vi "AO_equations_to_waveform.vi"(5 "variable/parameter names":string[](array[string]), 7 "minimum/current values":dbl[](array[numeric]), 8 "error in (no error)":errorcluster, 9 "Samples per second":dbl, 10 "Total AO Time":string, 11 "Analog Output Equations for each Channel":string[](array[string])) -> (0 "error out":errorcluster, 2 "Total # Samples":i32, 3 "Waveform Graph":waveform(dbl)[](graph))   [LabVIEW 2013]
uses:
  <vilib>/gmath/NI_Gmath.lvlib
  <vilib>/measure/NI_MAPro.lvlib
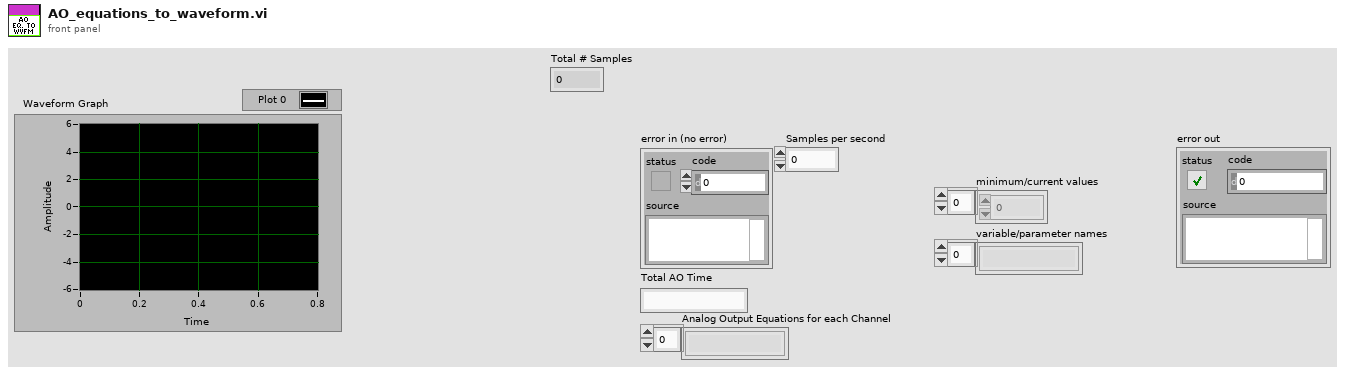
[diagram p1: front panel]
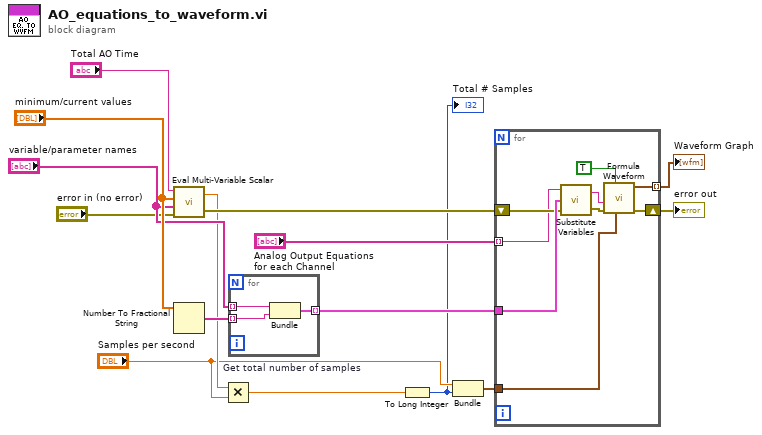
[diagram p0: block diagram]
diagram:
  n1 = call <vilib>:"Eval Multi-Variable Scalar.vi"("error in (no error)"="error in (no error)", "Variables"="variable/parameter names", "X Values"="minimum/current values", "formula"="Total AO Time") -> ("error out"=w8:errorcluster, "y value"=w5:dbl)
  n2 = Number To Fractional String(number="minimum/current values") -> (F-format string=w15:string[])  [unwired: 3 in]
  n3 = Multiply "Get total number of samples"(x=w5, y="Samples per second") -> (x*y=w3:dbl)
  n4 = for {
    tunnel: "variable/parameter names" -> [w18] mode=indexing
    tunnel: w15 -> [w17] mode=indexing
    tunnel: [w16] -> w14 mode=indexing
    n5 = Bundle("Name (a,a0...a9)"=w18, "min"=w17) -> (w16:cluster{"Name (a,a0...a9)":string, "min":string})  [unwired: 1 in]
  }
  n6 = To Long Integer(number=w3) -> (32bit integer=w2:i32)
  "Total # Samples" <- w2
  n7 = Bundle("Samples per second"="Samples per second", w2) -> (w13:cluster{"Samples per second":dbl, i32})  [unwired: 1 in]
  n8 = for {
    tunnel: "Analog Output Equations for each Channel" -> [w22] mode=indexing
    tunnel: w14 -> [w27]
    shift-right: [w24] -> w6
    shift-left: w8 -> [w25]
    tunnel: w13 -> [w21]
    tunnel: [w19] -> w1 mode=indexing
    n9 = call <vilib>:"Substitute Variables.vi"("error in (no error)"=w25, "Substitution Rules"=w27, "original formula"=w22) -> ("error out"=w20:errorcluster, "formula after substitution"=w26:string)
    n10 = call <vilib>:"Formula Waveform.vi"("sampling info"=w21, "reset signal"=TRUE, "error in (no error)"=w20, "formula"=w26) -> ("error out"=w24:errorcluster, "signal out"=w19:waveform(dbl))  [unwired: 6 in]
  }
  "error out" <- w6
  "Waveform Graph" <- w1
